vi "clearpath_set_platform_time.vi"(0 "ClearpathComm":T1, 1 "New Time":u32) -> ()   [LabVIEW 2011, in "clearpath_interface.lvlib"]
doc: "Formats a Set Platform Time command (0x5) given an input time. Uses the onboard Clearpath library to perform the actual message formatting."
uses:
  clearpath_interface.lvlib
  IGVC 2013/Code/Project 1.0/Motors/Husky/cwrap_crio.dll
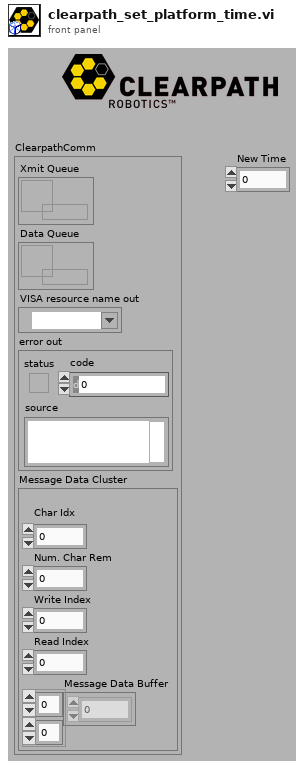
[diagram p1: front panel]
types:
  T1 = cluster{"Xmit Queue":refnum<queue>, "Data Queue":refnum<queue>, "VISA resource name out":refnum<visa-resource-name>, "error out":errorcluster, "Message Data Cluster":cluster{"\nChar Idx":u8, "Num. Char Rem":u8, "Write Index":u8, "Read Index":u8, "Message Data Buffer":u8[][]}}
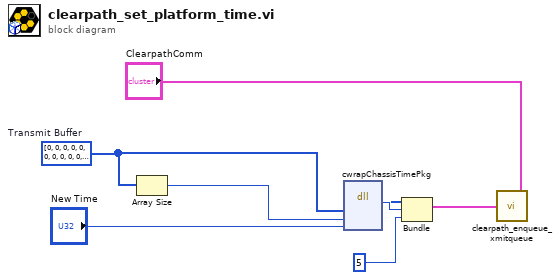
[diagram p0: block diagram]
diagram:
  w5 = u8[] [0, 0, 0, 0, 0, 0, 0, 0, 0, 0, 0, 0, 0, 0, 0, 0, 0, 0, 0, 0, 0, 0, 0, 0, 0, 0, 0, 0, 0, 0, 1, 0, 0, 0, 5]  # Transmit Buffer
  n1 = Array Size(array=w5) -> (size(s)=w6:i32)
  n2 = dll-call lib="C:/Users/whitemrj/Documents/GitHub/IGVC/IGVC 2013/Code/Project 1.0/Motors/Husky/cwrap_crio.dll" fn="cwrapChassisTimePkg"("buf"=w5, "buf_size"=w6, "time"="New Time") -> ("return type"=w8:i32, "buf"=w7:u8[])  [unwired: 5 in, 2 out]
  n3 = Bundle("buf"=w7, "return type"=w8, 5) -> (w2:cluster{"buf":u8[], "return type":i32, i32})  [unwired: 1 in]
  n4 = call "clearpath_enqueue_xmitqueue.vi"("ClearpathComm"="ClearpathComm", "Cluster"=w2) -> ()
